vi "RemainingRT_us.vi"(7 "Time period target":i32 caption="Time period target [µs]", 11 "Error in":errorcluster caption="Error in (no error)", 12 "Start time in":i64=-1 caption="Start time in (-1: init) [µs]" min=-1 max=4294967295) -> (8 "Remaining time":i32 caption="Remaining time [µs]", 10 "Elapsed time":i32 caption="Elapsed time [µs]", 13 "Now":i64 caption="Now [µs]", 14 "Start time out":i64 caption="Start time out [µs]", 15 "Error out":errorcluster)   [LabVIEW 2017, in "GPTiming.lvlib"]
doc: "Calculates <B>Remaining time</B> of <B>Time period target</B> since <B>Start time in</B>.\n\n<B>Start time in</B> will be returned in <B>Start time out</B>. Set <B>Start time in</B> to -1 (or leave it unwired) to get the current time returned in <B>Start time out</B> instead. <B>Now</B> will always be the current time.\n\nThis VI uses the Real-Time microsecond tick counter and will be able to count for 2^31-1 microseconds (almost 36 minutes) before <B>Remaining time</B> wraps around. <B>Remaining time</B> will be latched at 0 from when the remaining time runs out and until the tick counter wraps around. <B>Elapsed time</B> will continue counting up past the remaining time running out, thus you can use this output to see how late you were if you overshoot the <B>Time period target</B>.\n\nThis VI is inlined. <B>Error in</B> is wired straight through to <B>Error out</B> to enable optional dataflow dependency (offering control of when <B>Now</B> is).\n\nSteen Schmidt\nGPower\n6/12 2013"
uses:
  GPTiming.lvlib
panel:
  # "Copyright © 2013\nGPower\nSee enclosed license file for terms and conditions"
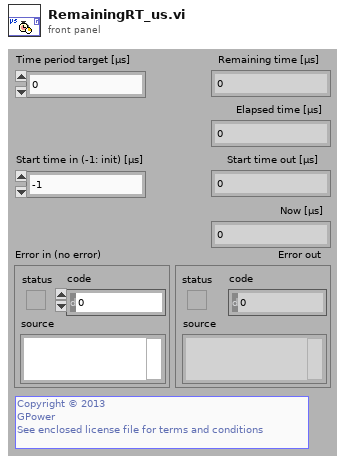
[diagram p1: front panel]
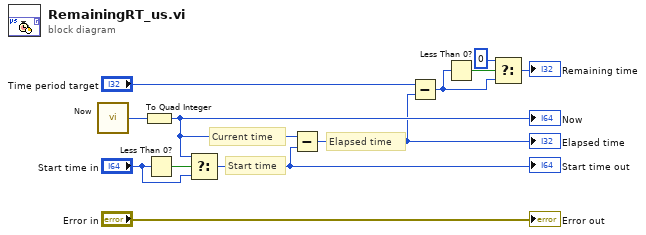
[diagram p0: block diagram]
diagram:
  # "Elapsed time"
  # "Current time"
  # "Start time"
  n1 = call "Now"() -> ("Tick Count(uSec)"=w2:u32)
  n2 = To Quad Integer(1:w2) -> (0:w8:i64)
  "Now" <- w8
  n3 = Less Than 0?(x="Start time in") -> (x < 0?=w11:bool)
  n4 = Select(t=w8, s=w11, f="Start time in") -> (s? t:f=w9:i64)
  "Start time out" <- w9
  n5 = Subtract(x=w8, y=w9) -> (x-y=w1:i64)
  "Elapsed time" <- w1
  n6 = Subtract(x="Time period target", y=w1) -> (x-y=w4:i64)
  n7 = Less Than 0?(x=w4) -> (x < 0?=w5:bool)
  n8 = Select(t=i64 0, s=w5, f=w4) -> (s? t:f=→"Remaining time":i64)
  "Error out" <- "Error in"
